vi "Shutdown.vi"(8 "error in (no error)":errorcluster, 11 "DAQ_QPT_Throlab in":refnum<class "DAQ_QPT_Throlab.lvclass">) -> (0 "error out":errorcluster, 3 "DAQ_QPT_Throlab out":refnum<class "DAQ_QPT_Throlab.lvclass">)   [LabVIEW 2020, in "DAQ_QPT_Throlab.lvlib" / "DAQ_QPT_Throlab.lvclass"]
uses:
  DAQ_QPT_Throlab.lvclass
  HAL Layer/Component/DAQ/DAQ/DAQ.lvclass
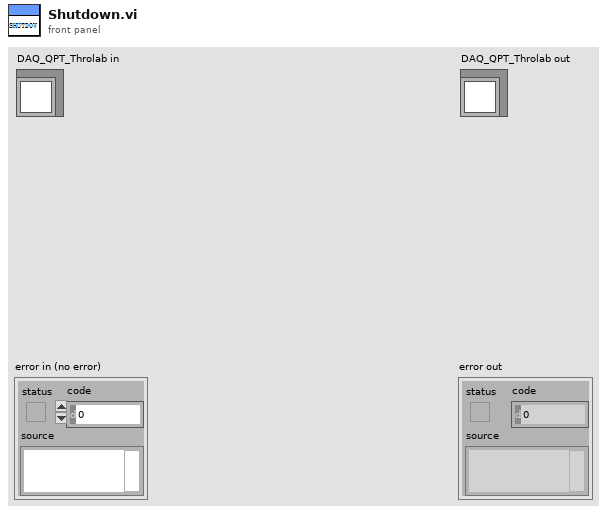
[diagram p1: front panel]
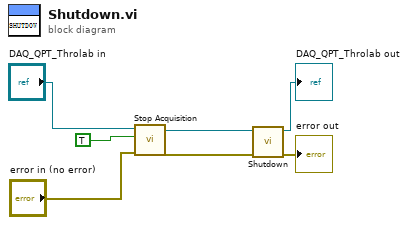
[diagram p0: block diagram]
diagram:
  n1 = call-dynamic "Stop Acquisition.vi"("error in (no error)"="error in (no error)", "Stop"=TRUE, "DAQ in"="DAQ_QPT_Throlab in") -> ("error out"=w4:errorcluster, "DAQ out"=w2:refnum<class "DAQ_QPT_Throlab.lvclass">)  [unwired: 7 in]
  n2 = call-parent "Shutdown.vi"("error in (no error)"=w4, "Device in"=w2) -> ("error out"=→"error out":errorcluster, "Device out"=→"DAQ_QPT_Throlab out":refnum<class "DAQ_QPT_Throlab.lvclass">)  [unwired: 8 in]
